vi "Pre-Build Action.vi"(6 "Top Level/Always Included VIs":path[](array[path]), 7 "Main Destination Path":path, 9 "Target Name":string, 10 "Build Specification Name":string, 11 "Project Path":path) -> (0 "error out":errorcluster)   [LabVIEW 2023]
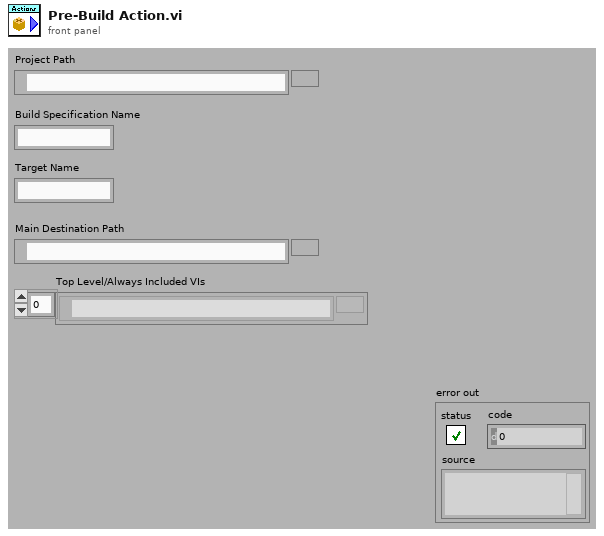
[diagram p1: front panel]
types:
  T1 = enum32{"Invalid", "Standard", "Closed", "Hidden", "Minimized", "Maximized"}
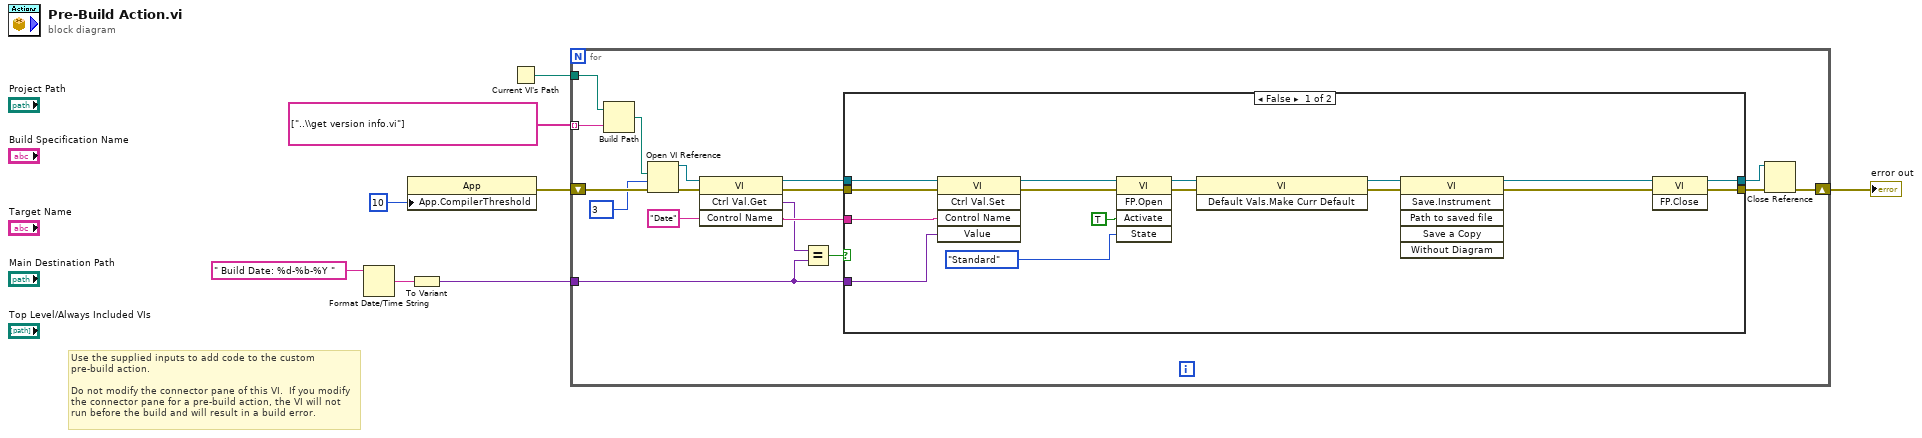
[diagram p0: block diagram]
diagram:
  # "Use the supplied inputs to add code to the custom pre-build action.\n\nDo not modify the connector pane of this VI.  If you modify the connector pane for a pre-build action, the VI will not run before the build and will result in a build error."
  n1 = Format Date/Time String(time format string (%c)=" Build Date: %d-%b-%Y ") -> (date/time string=w6:string)  [unwired: 2 in]
  n2 = property class="App"("App.CompilerThreshold"=u32 10 ("Application:Compiler Threshold")) -> (error out=w4:errorcluster)  [unwired: 2 in, 1 out]
  n3 = To Variant(anything=w6) -> (Variant=w5:variant)
  n4 = Current VI's Path() -> (path=w2:path)
  n5 = for {
    tunnel: string[] ["..\\get version info.vi"] -> [w22] mode=indexing
    shift-right: [w24] -> w1
    shift-left: w4 -> [w23]
    tunnel: w5 -> [w9]
    tunnel: w2 -> [w20]
    w12 = "Date" ("Control Name")
    n6 = Build Path(base path=w20, name or relative path=w22) -> (appended path=w21:path)
    n7 = Open VI Reference(vi path=w21, options=3, error in (no error)=w23) -> (vi reference=w16:refnum<vi>, error out=w14:errorcluster)  [unwired: 3 in]
    n8 = invoke class="VI" method="Ctrl Val.Get"(reference=w16, error in=w14, "Control Name"=w12) -> (reference out=w15:refnum<vi>, error out=w13:errorcluster, "Get Control Value Variant"=w11:variant)  [unwired: 1 in, 1 out]
    n9 = Equal?(x=w11, y=w9) -> (x = y?=w10:bool)
    n10 = case shown="False" w10 {
      tunnel: [w33 w42] -> w19
      tunnel: [w31 w41] -> w18
      tunnel: w15 -> [w29 w42]
      tunnel: w13 -> [w28 w41]
      tunnel: w12 -> [w27 _]
      tunnel: w9 -> [w26 _]
      frame False {
        n11 = invoke class="VI" method="Ctrl Val.Set"(reference=w29, error in=w28, "Control Name"=w27, "Value"=w26) -> (reference out=w39:refnum<vi>, error out=w37:errorcluster)  [unwired: 1 in, 3 out]
        n12 = invoke class="VI" method="FP.Open"(reference=w39, error in=w37, "Activate"=TRUE ("Activate?"), "State"=T1."Standard") -> (reference out=w38:refnum<vi>, error out=w36:errorcluster)  [unwired: 1 in, 3 out]
        n13 = invoke class="VI" method="Default Vals.Make Curr Default"(reference=w38, error in=w36) -> (reference out=w30:refnum<vi>, error out=w40:errorcluster)  [unwired: 1 in, 1 out]
        n14 = invoke class="VI" method="Save.Instrument"(reference=w30, error in=w40) -> (reference out=w34:refnum<vi>, error out=w32:errorcluster)  [unwired: 4 in, 4 out]
        n15 = invoke class="VI" method="FP.Close"(reference=w34, error in=w32) -> (reference out=w33:refnum<vi>, error out=w31:errorcluster)  [unwired: 1 in, 1 out]
      }
      frame True {
      }
    }
    n16 = Close Reference(reference=w19, error in (no error)=w18) -> (error out=w24:errorcluster)
  }
  "error out" <- w1
